vi "Helper - Check for irons.vi"(9 "Angle to check":dbl, 10 "Wind - Irons range":dbl, 11 "Wind + Irons range":dbl) -> (2 "In irons?":bool)   [LabVIEW 2011]
doc: "Takes in wind angle + irons range and wind angle - irons range, both normalized to be within 0-360, and checks whether the angle inputed falls within the irons range."
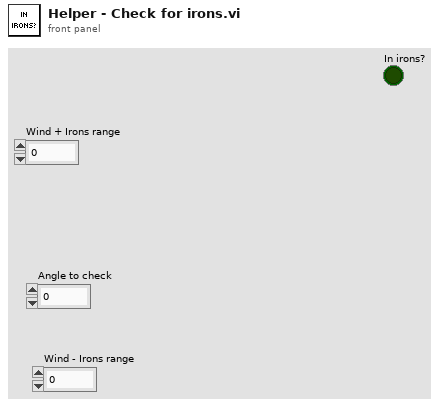
[diagram p1: front panel]
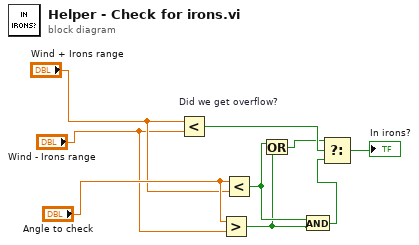
[diagram p0: block diagram]
diagram:
  n1 = Less? "Did we get overflow?"(x="Wind + Irons range", y="Wind - Irons range") -> (x < y?=w9:bool)
  n2 = Greater?(x="Angle to check", y="Wind - Irons range") -> (0:w5:bool)
  n3 = Less?(x="Angle to check", y="Wind + Irons range") -> (x < y?=w6:bool)
  n4 = Or(x=w6, y=w5) -> (x .or. y?=w8:bool)
  n5 = And(x=w6, y=w5) -> (x .and. y?=w7:bool)
  n6 = Select(t=w8, s=w9, f=w7) -> (s? t:f=→"In irons?":bool)
